vi "alpha_0.5.vi"() -> ()   [LabVIEW 2018]
panel:
  in  "func":string
  in  "Path":path
  out "Congestionamento 2":bool
  in  "Rácio de entrada 2":dbl
  in  "Slide 2":dbl(slide) scale=0.0..10.0
  in  "Velocidade 2":dbl
  out "Vel3":bool
  out "Vel2":bool
  out "Vel1":bool
  out "RP1 3":bool
  out "GP1 3":bool
  out "G1 3":bool
  out "Y1 3":bool
  out "R1 3":bool
  out "RP1 2":bool
  out "GP1 2":bool
  out "G1 2":bool
  out "Y1 2":bool
  out "R1 2":bool
  out "RP1":bool
  out "GP1":bool
  out "G1":bool
  out "Y1":bool
  out "R1":bool
  in  "Rácio de entrada":dbl
  in  "Rácio de entrada 3":dbl
  out "Tempo no Vermelho":dbl caption="Elapsed Time (s)"
  out "Tempo no Verde + Amarelo":dbl caption="Elapsed Time (s)"
  out "Congestionamento 3":bool
  out "Congestionamento 1":bool
  in  "Slide 3":dbl(slide) scale=0.0..10.0
  in  "Slide 1":dbl(slide) scale=0.0..10.0
  in  "Caso de emergência":bool
  out "GreenP 2":bool
  out "RedP 2":bool
  out "GreenP 1":bool
  out "RedP 1":bool
  in  "Estado 2":dbl
  out "Velocidade excedida 3":bool
  in  "Velocidade 3":dbl
  out "RED 4":bool
  out "YELLOW 4":bool
  out "GREEN 4":bool
  out "Velocidade excedida 2":bool
  in  "Velocidade":dbl
  out "RED 3":bool
  out "YELLOW 3":bool
  out "GREEN 3":bool
  in  "stop":bool
  in  "Timer (s)":dbl
  # "Inputs"
  # "Inputs"
  # "Inputs"
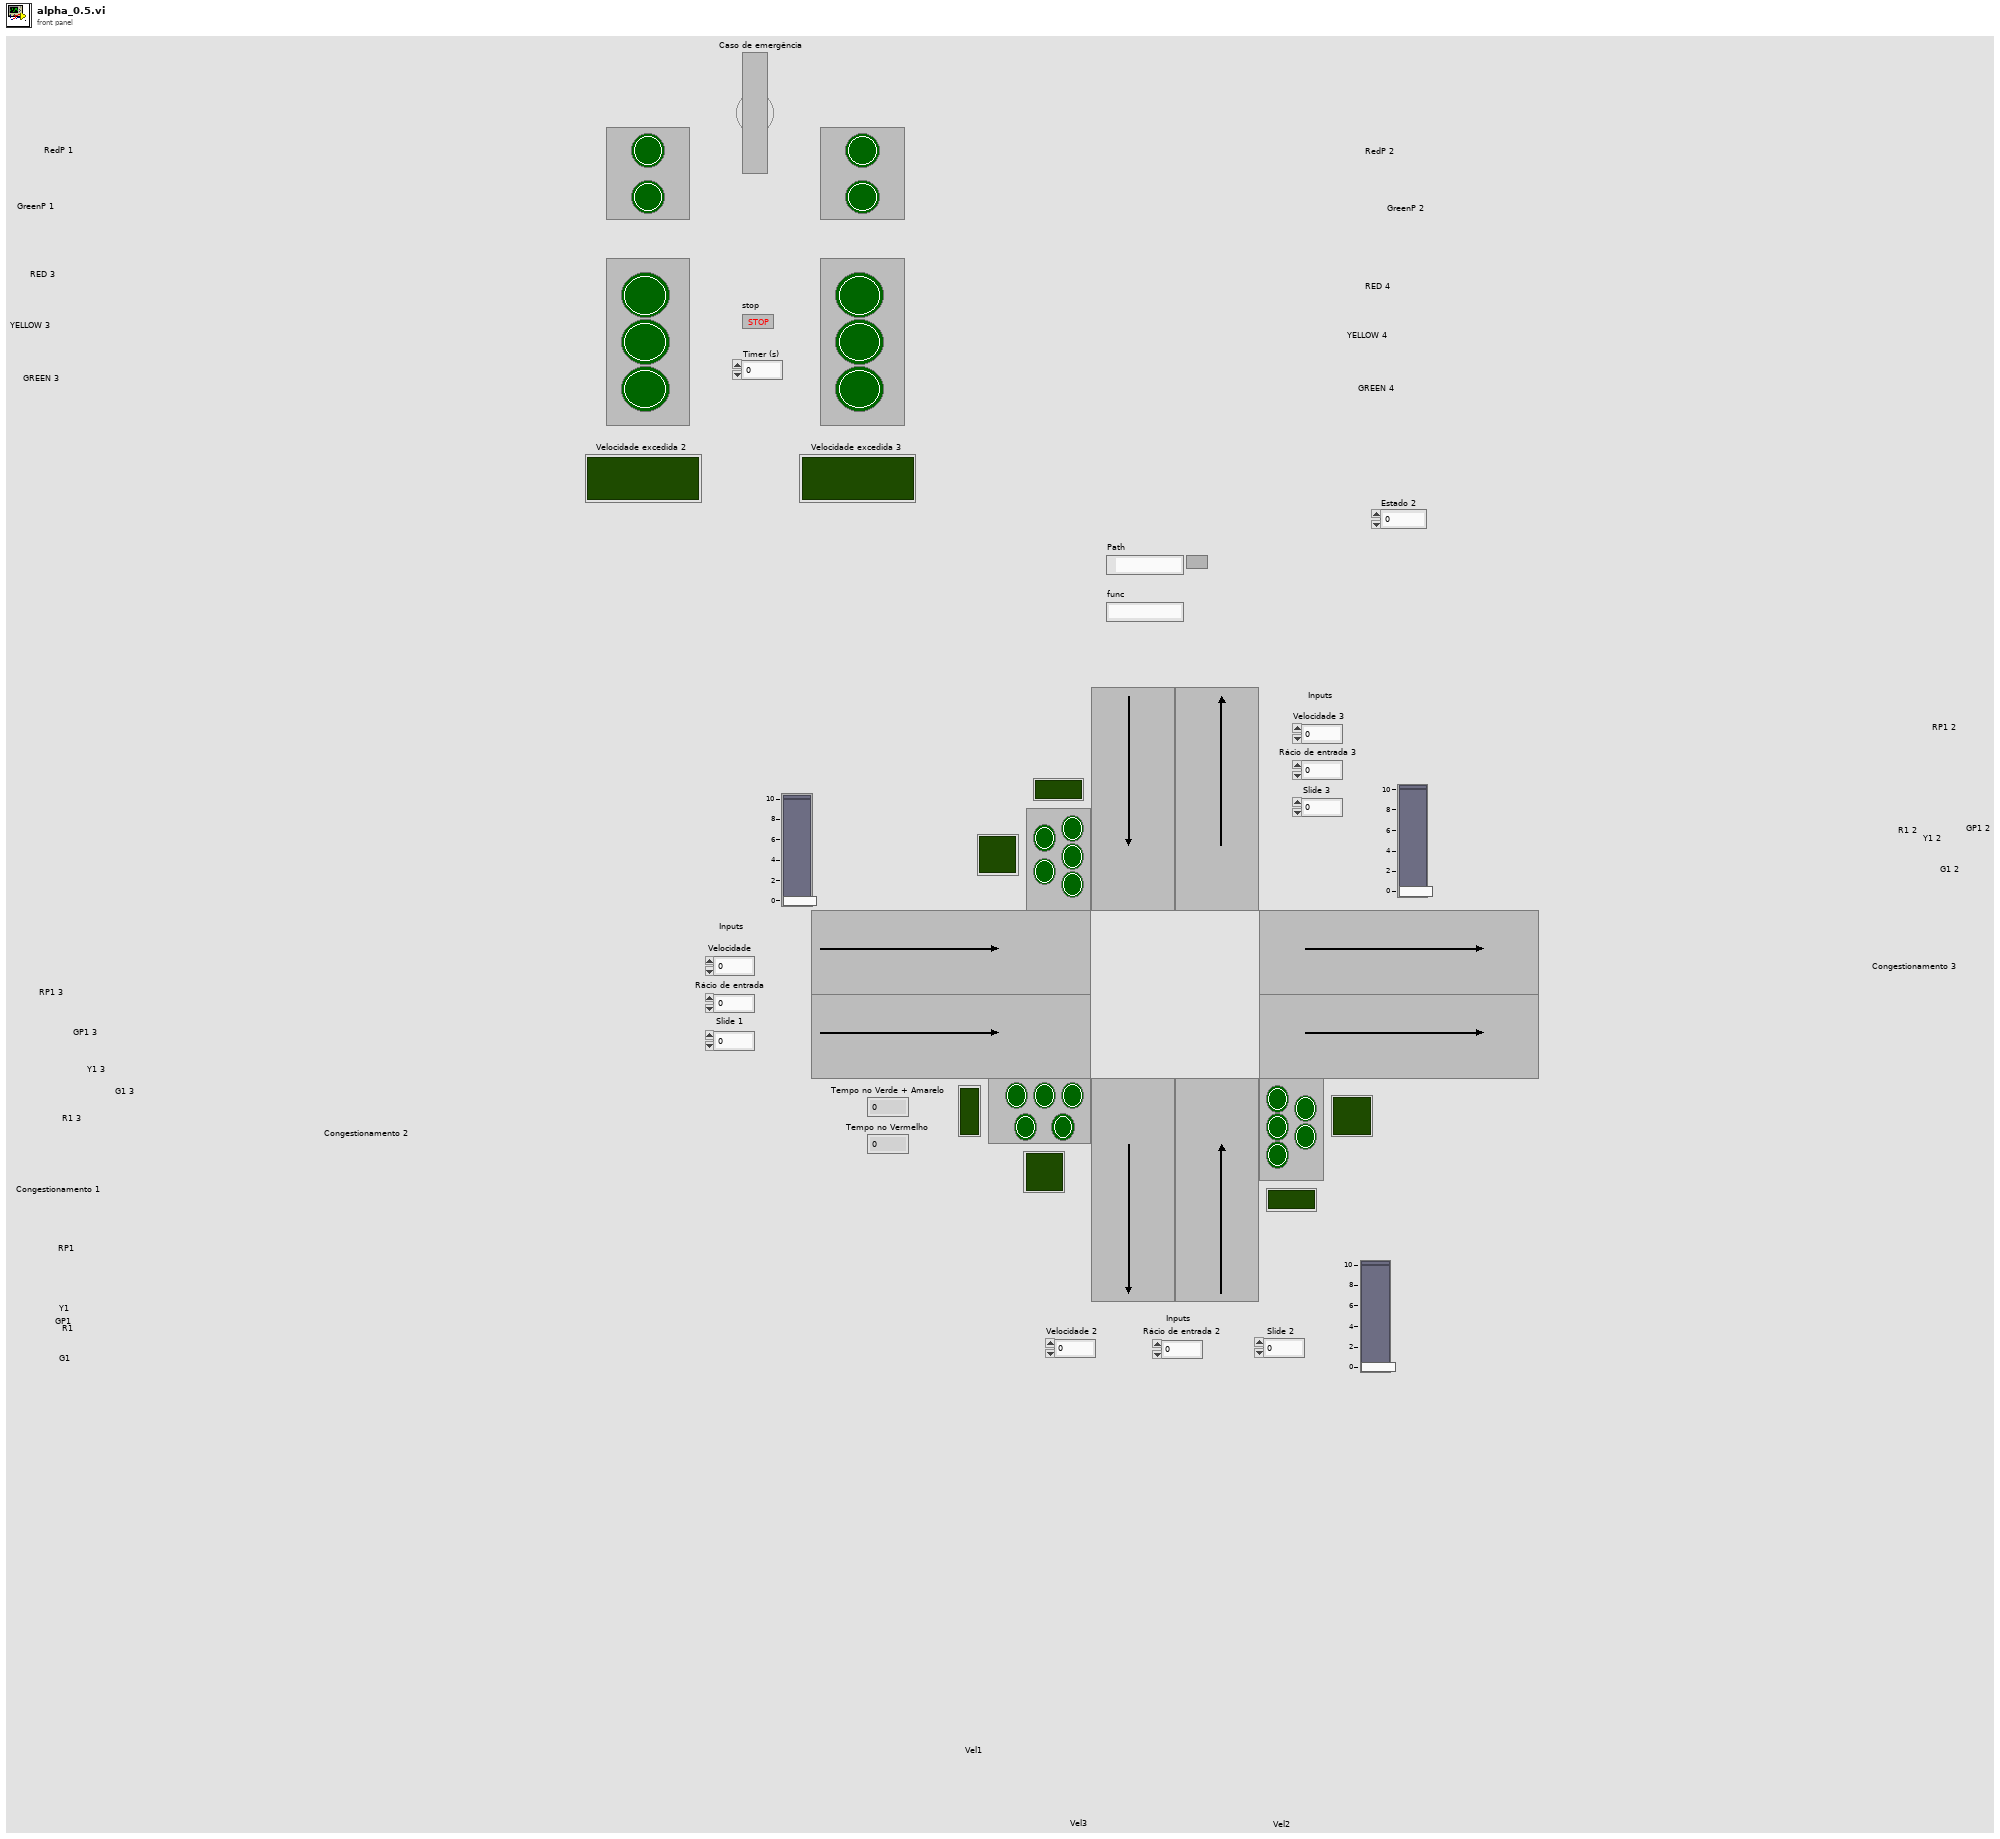
[diagram p1: front panel]
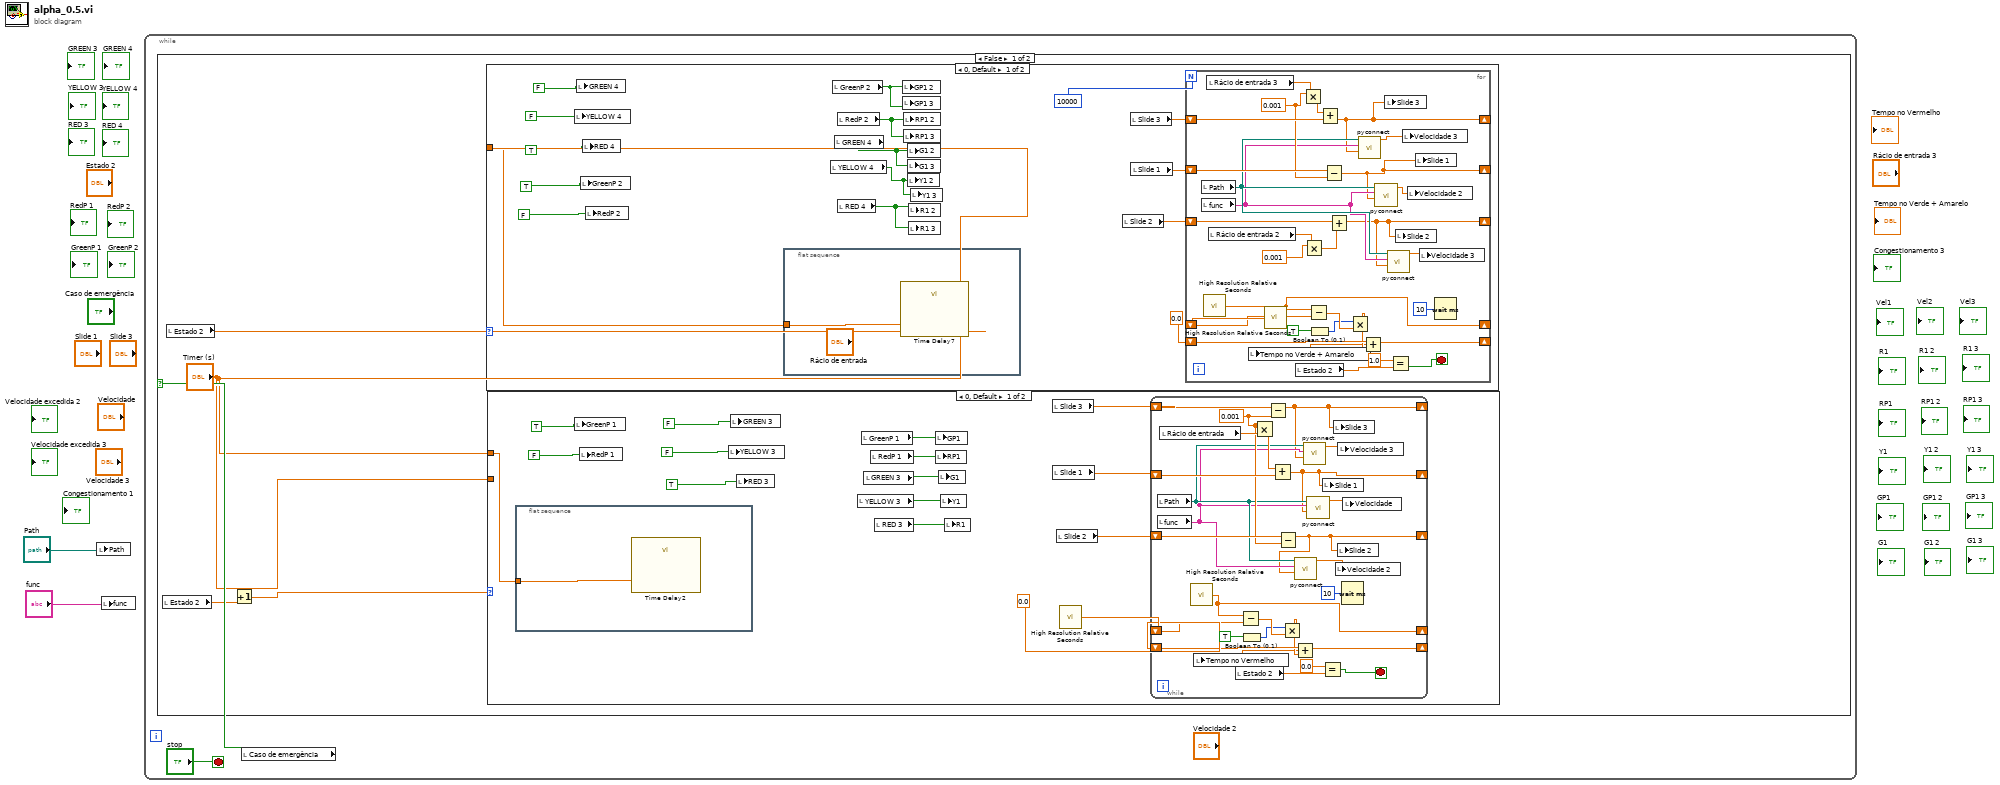
[diagram p0: block diagram]
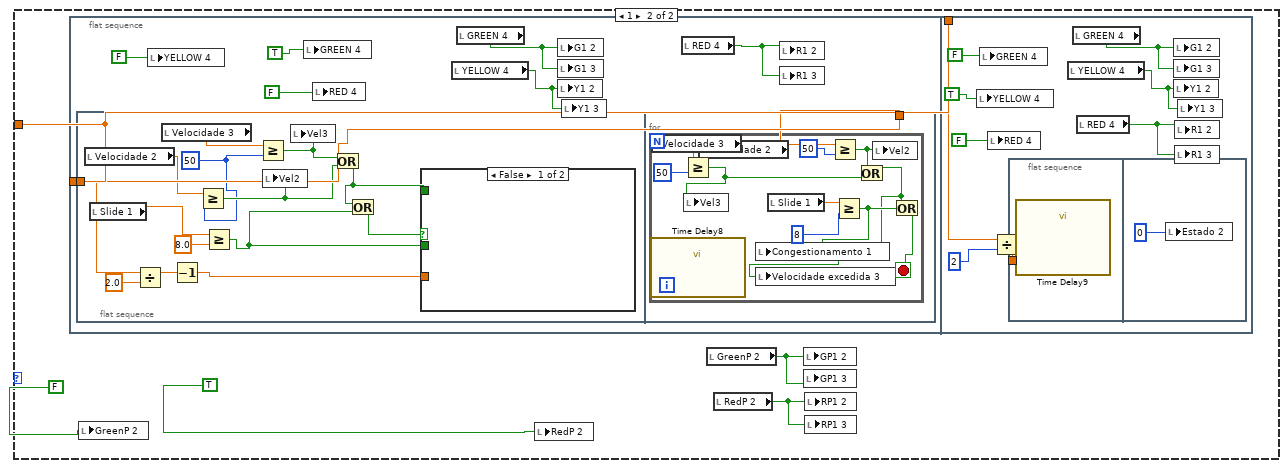
[diagram p2: hidden frame]
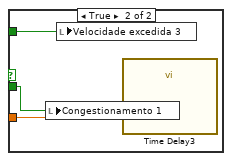
[diagram p3: hidden frame]
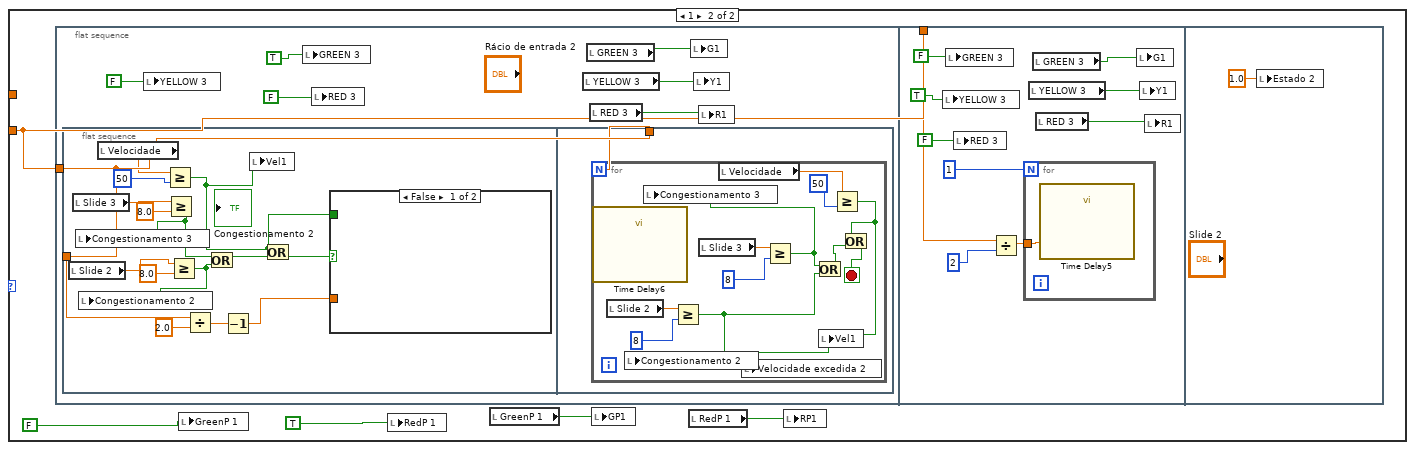
[diagram p4: hidden frame]
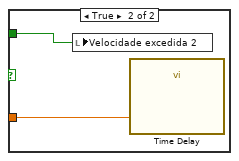
[diagram p5: hidden frame]
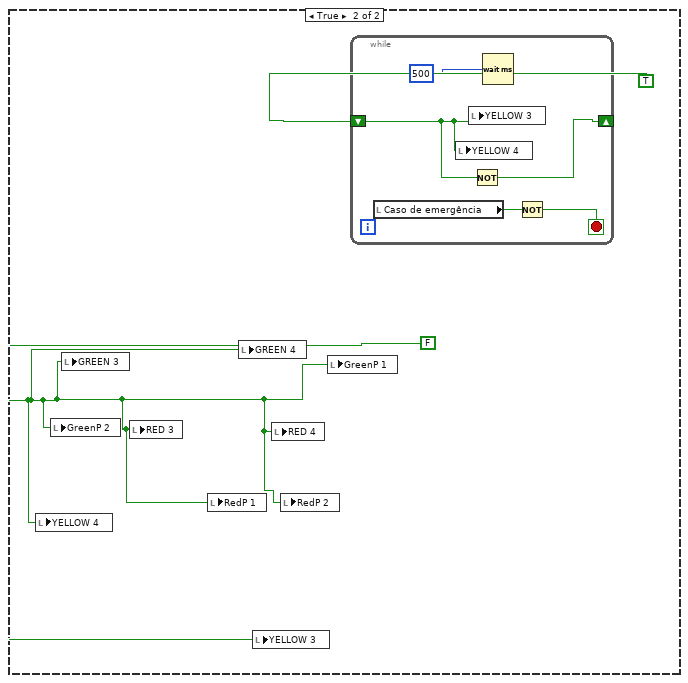
[diagram p6: hidden frame]
diagram:
  n1 = local write "Path"("Path") -> ()
  n2 = local write "func"("func") -> ()
  n3 = while {
    stop <- "stop" stop-if-true
    n4 = local read "Caso de emergência"() -> (w3:bool)
    n5 = case shown="False" w3 {
      frame False {
        n6 = local read "Estado 2"() -> (w8:dbl)
        n7 = local read "Estado 2"() -> (w6:dbl)
        n8 = Increment(x=w8) -> (x+1=w7:dbl)
        n9 = case shown="0, Default" w6 {
          tunnel: "Timer (s)" -> [w20 w60]
          frame 0, Default {
            n10 = local write "YELLOW 4"(FALSE) -> ()
            n11 = local write "GREEN 4"(FALSE) -> ()
            n12 = local write "GreenP 2"(TRUE) -> ()
            n13 = local write "RED 4"(TRUE) -> ()
            n14 = local write "RedP 2"(FALSE) -> ()
            n15 = flat-sequence {
              tunnel: w20 -> [w55]
              frame #0 {
                n16 = call "Time Delay7"("Delay Time (s)"=w55) -> ()  [unwired: 10 in, 1 out]
              }
            }
            n17 = local read "YELLOW 4"() -> (w11:bool)
            n18 = local read "GreenP 2"() -> (w14:bool)
            n19 = local read "GREEN 4"() -> (w12:bool)
            n20 = local read "RedP 2"() -> (w13:bool)
            n21 = local read "RED 4"() -> (w10:bool)
            n22 = local write "GP1 2"(w14) -> ()
            n23 = local write "GP1 3"(w14) -> ()
            n24 = local write "RP1 2"(w13) -> ()
            n25 = local write "RP1 3"(w13) -> ()
            n26 = local write "G1 2"(w12) -> ()
            n27 = local write "G1 3"(w12) -> ()
            n28 = local write "Y1 2"(w11) -> ()
            n29 = local write "R1 2"(w10) -> ()
            n30 = local write "R1 3"(w10) -> ()
            n31 = local write "Y1 3"(w11) -> ()
            n32 = local read "Slide 2"() -> (w9:dbl)
            n33 = local read "Slide 3"() -> (w15:dbl)
            n34 = local read "Slide 1"() -> (w16:dbl)
            n35 = call <vilib>:"High Resolution Relative Seconds.vi"() -> ("relative seconds"=w19:dbl)
            n36 = for {
              N: 10000 -> [_]
              shift-right: [w52] -> _
              shift-left: w19 -> [w53]
              shift-right: [w46] -> _
              shift-left: 0.0 -> [w51]
              shift-right: [w31] -> _
              shift-left: w15 -> [w42]
              shift-right: [w30] -> _
              shift-left: w16 -> [w39]
              shift-right: [w29] -> _
              shift-left: w9 -> [w37]
              stop <- w44 stop-if-true
              w38 = 0.001 ("x")
              n37 = local read "Path"() -> (w33:path)
              n38 = local read "func"() -> (w32:string)
              n39 = call <vilib>:"High Resolution Relative Seconds.vi"() -> ("relative seconds"=w52:dbl)
              n40 = local read "Rácio de entrada 3"() -> (w41:dbl)
              n41 = local read "Rácio de entrada 2"() -> (w35:dbl)
              n42 = local read "Estado 2"() -> (w45:dbl)
              n43 = Multiply(x=w38, y=w41) -> (x*y=w40:dbl)
              n44 = Multiply(x=0.001, y=w35) -> (x*y=w34:dbl)
              n45 = Subtract(x=w52, y=w53) -> (x-y=w49:dbl)
              n46 = Boolean To (0,1)(Boolean=TRUE) -> (0, 1=w47:i16)
              n47 = Add(x=w40, y=w42) -> (x+y=w31:dbl)
              n48 = Subtract(x=w39, y=w38) -> (x-y=w30:dbl)
              n49 = Add(x=w37, y=w34) -> (x+y=w29:dbl)
              n50 = Multiply(x=w47, y=w49) -> (x*y=w48:dbl)
              n51 = call "pyconnect.vi"("slider"=w31, "function name"=w32, "module path"=w33) -> ("Numeric"=w28:dbl)  [unwired: 8 in]
              n52 = Add(x=w51, y=w48) -> (x+y=w46:dbl)
              n53 = local write "Tempo no Verde + Amarelo"(w46) -> ()
              n54 = call "pyconnect.vi"("slider"=w30, "function name"=w32, "module path"=w33) -> ("Numeric"=w27:dbl)  [unwired: 8 in]
              n55 = local write "Slide 3"(w31) -> ()
              n56 = call "pyconnect.vi"("slider"=w29, "function name"=w32, "module path"=w33) -> ("Numeric"=w26:dbl)  [unwired: 8 in]
              n57 = Equal?(x=1.0, y=w45) -> (x = y?=w44:bool)
              n58 = local write "Slide 2"(w29) -> ()
              n59 = local write "Velocidade 3"(w28) -> ()
              n60 = local write "Velocidade 2"(w27) -> ()
              n61 = local write "Slide 1"(w30) -> ()
              n62 = local write "Velocidade 3"(w26) -> ()
              n63 = Wait (ms)(milliseconds to wait=u32 10) -> ()  [unwired: 1 out]
            }
          }
          frame 1 {
            n64 = flat-sequence {
              tunnel: w60 -> [w64]
              tunnel: w60 -> [w101]
              frame #0 {
                n65 = flat-sequence {
                  tunnel: w64 -> [w77]
                  tunnel: w64 -> [w85]
                  frame #0 {
                    w68 = 50
                    n66 = local read "Velocidade 2"() -> (w70:dbl)
                    n67 = local read "Slide 1"() -> (w74:dbl)
                    n68 = Divide(x=w77, y=2.0) -> (x/y=w80:dbl)
                    n69 = local read "Velocidade 3"() -> (w79:dbl)
                    n70 = Decrement(x=w80) -> (x-1=w81:dbl)
                    n71 = Greater Or Equal?(x=w70, y=w68) -> (x >= y?=w69:bool)
                    n72 = Greater Or Equal?(x=w74, y=8.0) -> (x >= y?=w72:bool)
                    n73 = Greater Or Equal?(x=w79, y=w68) -> (x >= y?=w73:bool)
                    n74 = local write "Vel2"(w69) -> ()
                    n75 = local write "Vel3"(w73) -> ()
                    n76 = Or(x=w73, y=w69) -> (x .or. y?=w71:bool)
                    n77 = Or(x=w71, y=w72) -> (x .or. y?=w75:bool)
                    n78 = case shown="False" w75 {
                      tunnel: w81 -> [_ w84]
                      tunnel: w71 -> [_ w82]
                      tunnel: w72 -> [_ w83]
                      frame False {
                      }
                      frame True {
                        n79 = local write "Congestionamento 1"(w83) -> ()
                        n80 = local write "Velocidade excedida 3"(w82) -> ()
                        n81 = call "Time Delay3"("Delay Time (s)"=w84) -> ()  [unwired: 10 in, 1 out]
                      }
                    }
                  }
                  frame #1 {
                    n82 = for {
                      N: w85 -> [_]
                      stop <- w94 stop-if-true
                      n83 = call "Time Delay8"() -> ()  [unwired: 11 in, 1 out]
                      n84 = local read "Velocidade 3"() -> (w96:dbl)
                      n85 = Greater Or Equal?(x=w96, y=50) -> (x >= y?=w90:bool)
                      n86 = local write "Vel3"(w90) -> ()
                      n87 = local read "Velocidade 2"() -> (w88:dbl)
                      n88 = local read "Slide 1"() -> (w93:dbl)
                      n89 = Greater Or Equal?(x=w88, y=50) -> (x >= y?=w86:bool)
                      n90 = Greater Or Equal?(x=w93, y=8) -> (x >= y?=w91:bool)
                      n91 = local write "Congestionamento 1"(w91) -> ()
                      n92 = Or(x=w86, y=w90) -> (x .or. y?=w89:bool)
                      n93 = local write "Velocidade excedida 3"(w89) -> ()
                      n94 = local write "Vel2"(w86) -> ()
                      n95 = Or(x=w89, y=w91) -> (x .or. y?=w94:bool)
                    }
                  }
                }
                n96 = local write "YELLOW 4"(FALSE) -> ()
                n97 = local write "GREEN 4"(TRUE) -> ()
                n98 = local write "RED 4"(FALSE) -> ()
                n99 = local read "YELLOW 4"() -> (w62:bool)
                n100 = local read "GREEN 4"() -> (w63:bool)
                n101 = local write "G1 2"(w63) -> ()
                n102 = local write "G1 3"(w63) -> ()
                n103 = local write "Y1 2"(w62) -> ()
                n104 = local write "Y1 3"(w62) -> ()
                n105 = local read "RED 4"() -> (w61:bool)
                n106 = local write "R1 2"(w61) -> ()
                n107 = local write "R1 3"(w61) -> ()
              }
              frame #1 {
                n108 = local write "YELLOW 4"(TRUE) -> ()
                n109 = local write "GREEN 4"(FALSE) -> ()
                n110 = local write "RED 4"(FALSE) -> ()
                n111 = Divide(x=w101, y=2) -> (x/y=w100:dbl)
                n112 = flat-sequence {
                  tunnel: w100 -> [w106]
                  frame #0 {
                    n113 = call "Time Delay9"("Delay Time (s)"=w106) -> ()  [unwired: 10 in, 1 out]
                  }
                  frame #1 {
                    n114 = local write "Estado 2"(0) -> ()
                  }
                }
                n115 = local read "YELLOW 4"() -> (w98:bool)
                n116 = local read "GREEN 4"() -> (w99:bool)
                n117 = local read "RED 4"() -> (w97:bool)
                n118 = local write "G1 2"(w99) -> ()
                n119 = local write "G1 3"(w99) -> ()
                n120 = local write "Y1 2"(w98) -> ()
                n121 = local write "R1 2"(w97) -> ()
                n122 = local write "R1 3"(w97) -> ()
                n123 = local write "Y1 3"(w98) -> ()
              }
            }
            n124 = local write "GreenP 2"(FALSE) -> ()
            n125 = local write "RedP 2"(TRUE) -> ()
            n126 = local read "GreenP 2"() -> (w57:bool)
            n127 = local read "RedP 2"() -> (w56:bool)
            n128 = local write "GP1 2"(w57) -> ()
            n129 = local write "GP1 3"(w57) -> ()
            n130 = local write "RP1 2"(w56) -> ()
            n131 = local write "RP1 3"(w56) -> ()
          }
        }
        n132 = case shown="0, Default" w7 {
          tunnel: "Timer (s)" -> [_ w153]
          tunnel: "Timer (s)" -> [w115 _]
          frame 0, Default {
            n133 = flat-sequence {
              tunnel: w115 -> [w124]
              frame #0 {
                n134 = call "Time Delay2"("Delay Time (s)"=w124) -> ()  [unwired: 10 in, 1 out]
              }
            }
            n135 = local write "GreenP 1"(TRUE) -> ()
            n136 = local write "RedP 1"(FALSE) -> ()
            n137 = local write "YELLOW 3"(FALSE) -> ()
            n138 = local write "GREEN 3"(FALSE) -> ()
            n139 = local write "RED 3"(TRUE) -> ()
            n140 = local read "YELLOW 3"() -> (w110:bool)
            n141 = local read "GreenP 1"() -> (w113:bool)
            n142 = local read "GREEN 3"() -> (w111:bool)
            n143 = local read "RedP 1"() -> (w112:bool)
            n144 = local read "RED 3"() -> (w109:bool)
            n145 = local write "GP1"(w113) -> ()
            n146 = local write "RP1"(w112) -> ()
            n147 = local write "G1"(w111) -> ()
            n148 = local write "Y1"(w110) -> ()
            n149 = local write "R1"(w109) -> ()
            n150 = local read "Slide 3"() -> (w116:dbl)
            n151 = local read "Slide 1"() -> (w114:dbl)
            n152 = local read "Slide 2"() -> (w108:dbl)
            n153 = call <vilib>:"High Resolution Relative Seconds.vi"() -> ("relative seconds"=w118:dbl)
            n154 = while {
              shift-right: [w148] -> _
              shift-left: w118 -> [w149]
              shift-right: [w142] -> _
              shift-left: 0.0 -> [w147]
              shift-right: [w128] -> _
              shift-left: w116 -> [w138]
              shift-right: [w129] -> _
              shift-left: w114 -> [w135]
              shift-right: [w130] -> _
              shift-left: w108 -> [w134]
              stop <- w140 stop-if-true
              w133 = 0.001 ("y")
              n155 = local read "Path"() -> (w132:path)
              n156 = local read "func"() -> (w131:string)
              n157 = local read "Rácio de entrada"() -> (w137:dbl)
              n158 = call <vilib>:"High Resolution Relative Seconds.vi"() -> ("relative seconds"=w148:dbl)
              n159 = local read "Estado 2"() -> (w141:dbl)
              n160 = Subtract(x=w148, y=w149) -> (x-y=w145:dbl)
              n161 = Boolean To (0,1)(Boolean=TRUE) -> (0, 1=w143:i16)
              n162 = Multiply(x=w133, y=w137) -> (x*y=w136:dbl)
              n163 = Subtract(x=w138, y=w133) -> (x-y=w128:dbl)
              n164 = Add(x=w136, y=w135) -> (x+y=w129:dbl)
              n165 = Subtract(x=w134, y=w133) -> (x-y=w130:dbl)
              n166 = Multiply(x=w143, y=w145) -> (x*y=w144:dbl)
              n167 = Add(x=w147, y=w144) -> (x+y=w142:dbl)
              n168 = local write "Tempo no Vermelho"(w142) -> ()
              n169 = call "pyconnect.vi"("slider"=w130, "function name"=w131, "module path"=w132) -> ("Numeric"=w125:dbl)  [unwired: 8 in]
              n170 = call "pyconnect.vi"("slider"=w128, "function name"=w131, "module path"=w132) -> ("Numeric"=w127:dbl)  [unwired: 8 in]
              n171 = call "pyconnect.vi"("slider"=w129, "function name"=w131, "module path"=w132) -> ("Numeric"=w126:dbl)  [unwired: 8 in]
              n172 = Equal?(x=0.0, y=w141) -> (x = y?=w140:bool)
              n173 = local write "Slide 1"(w129) -> ()
              n174 = local write "Slide 3"(w128) -> ()
              n175 = local write "Velocidade 2"(w125) -> ()
              n176 = local write "Slide 2"(w130) -> ()
              n177 = local write "Velocidade 3"(w127) -> ()
              n178 = Wait (ms)(milliseconds to wait=u32 10) -> ()  [unwired: 1 out]
              n179 = local write "Velocidade"(w126) -> ()
            }
          }
          frame 1 {
            n180 = flat-sequence {
              tunnel: w153 -> [w159]
              tunnel: w153 -> [w195]
              frame #0 {
                n181 = flat-sequence {
                  tunnel: w159 -> [w175]
                  tunnel: w159 -> [w180]
                  frame #0 {
                    n182 = local read "Slide 2"() -> (w163:dbl)
                    n183 = local read "Slide 3"() -> (w170:dbl)
                    n184 = local read "Velocidade"() -> (w177:dbl)
                    n185 = Greater Or Equal?(x=w177, y=50) -> (x >= y?=w168:bool)
                    n186 = Greater Or Equal?(x=w170, y=8.0) -> (x >= y?=w167:bool)
                    n187 = local write "Congestionamento 3"(w167) -> ()
                    n188 = Greater Or Equal?(x=w163, y=8.0) -> (x >= y?=w164:bool)
                    n189 = local write "Congestionamento 2"(w164) -> ()
                    n190 = Divide(x=w175, y=2.0) -> (x/y=w174:dbl)
                    n191 = Or(x=w167, y=w164) -> (x .or. y?=w166:bool)
                    n192 = Decrement(x=w174) -> (x-1=w172:dbl)
                    n193 = local write "Vel1"(w168) -> ()
                    n194 = Or(x=w168, y=w166) -> (x .or. y?=w171:bool)
                    n195 = case shown="False" w171 {
                      tunnel: w172 -> [_ w179]
                      tunnel: w168 -> [_ w178]
                      frame False {
                      }
                      frame True {
                        n196 = local write "Velocidade excedida 2"(w178) -> ()
                        n197 = call "Time Delay"("Delay Time (s)"=w179) -> ()  [unwired: 10 in, 1 out]
                      }
                    }
                  }
                  frame #1 {
                    n198 = for {
                      N: w180 -> [_]
                      stop <- w187 stop-if-true
                      n199 = call "Time Delay6"() -> ()  [unwired: 11 in, 1 out]
                      n200 = local read "Slide 2"() -> (w184:dbl)
                      n201 = Greater Or Equal?(x=w184, y=8) -> (x >= y?=w181:bool)
                      n202 = local write "Congestionamento 2"(w181) -> ()
                      n203 = local read "Slide 3"() -> (w189:dbl)
                      n204 = local read "Velocidade"() -> (w191:dbl)
                      n205 = Greater Or Equal?(x=w189, y=8) -> (x >= y?=w182:bool)
                      n206 = local write "Congestionamento 3"(w182) -> ()
                      n207 = Or(x=w182, y=w181) -> (x .or. y?=w183:bool)
                      n208 = Greater Or Equal?(x=w191, y=50) -> (x >= y?=w186:bool)
                      n209 = local write "Velocidade excedida 2"(w186) -> ()
                      n210 = local write "Vel1"(w186) -> ()
                      n211 = Or(x=w186, y=w183) -> (x .or. y?=w187:bool)
                    }
                  }
                }
                n212 = local write "YELLOW 3"(FALSE) -> ()
                n213 = local write "GREEN 3"(TRUE) -> ()
                n214 = local write "RED 3"(FALSE) -> ()
                n215 = local read "YELLOW 3"() -> (w157:bool)
                n216 = local read "GREEN 3"() -> (w158:bool)
                n217 = local read "RED 3"() -> (w156:bool)
                n218 = local write "G1"(w158) -> ()
                n219 = local write "Y1"(w157) -> ()
                n220 = local write "R1"(w156) -> ()
              }
              frame #1 {
                n221 = local write "YELLOW 3"(TRUE) -> ()
                n222 = local write "GREEN 3"(FALSE) -> ()
                n223 = local write "RED 3"(FALSE) -> ()
                n224 = Divide(x=w195, y=2) -> (x/y=w198:dbl)
                n225 = for {
                  N: 1 -> [_]
                  tunnel: w198 -> [w202]
                  n226 = call "Time Delay5"("Delay Time (s)"=w202) -> ()  [unwired: 10 in, 1 out]
                }
                n227 = local read "YELLOW 3"() -> (w194:bool)
                n228 = local read "GREEN 3"() -> (w192:bool)
                n229 = local read "RED 3"() -> (w193:bool)
                n230 = local write "G1"(w192) -> ()
                n231 = local write "Y1"(w194) -> ()
                n232 = local write "R1"(w193) -> ()
              }
              frame #2 {
                n233 = local write "Estado 2"(1.0 ("Estado 2")) -> ()
              }
            }
            n234 = local write "GreenP 1"(FALSE) -> ()
            n235 = local write "RedP 1"(TRUE) -> ()
            n236 = local read "GreenP 1"() -> (w151:bool)
            n237 = local write "GP1"(w151) -> ()
            n238 = local read "RedP 1"() -> (w152:bool)
            n239 = local write "RP1"(w152) -> ()
          }
        }
      }
      frame True {
        w204 = FALSE
        n240 = local write "YELLOW 4"(w204) -> ()
        n241 = local write "GreenP 2"(w204) -> ()
        n242 = local write "GREEN 3"(w204) -> ()
        n243 = local write "RED 3"(w204) -> ()
        n244 = local write "RedP 1"(w204) -> ()
        n245 = local write "GREEN 4"(w204) -> ()
        n246 = local write "YELLOW 3"(w204) -> ()
        n247 = local write "RED 4"(w204) -> ()
        n248 = local write "RedP 2"(w204) -> ()
        n249 = local write "GreenP 1"(w204) -> ()
        n250 = while {
          shift-right: [w210] -> _
          shift-left: TRUE -> [w206]
          stop <- w207 stop-if-true
          n251 = local read "Caso de emergência"() -> (w208:bool)
          n252 = local write "YELLOW 4"(w206) -> ()
          n253 = local write "YELLOW 3"(w206) -> ()
          n254 = Not(x=w206) -> (.not. x?=w210:bool)
          n255 = Wait (ms)(milliseconds to wait=500) -> ()  [unwired: 1 out]
          n256 = Not(x=w208) -> (.not. x?=w207:bool)
        }
      }
    }
  }
